vi "ParseRealTimeData.vi"(8 "error in (no error)":errorcluster, 11 "Raw Data":string) -> (0 "error out":errorcluster, 2 "BuySellBar":cluster{dbl[], dbl[]}[](graph), 3 "Price":T1)   [LabVIEW 2013]
uses:
  ctrl/TYPE Price.ctl
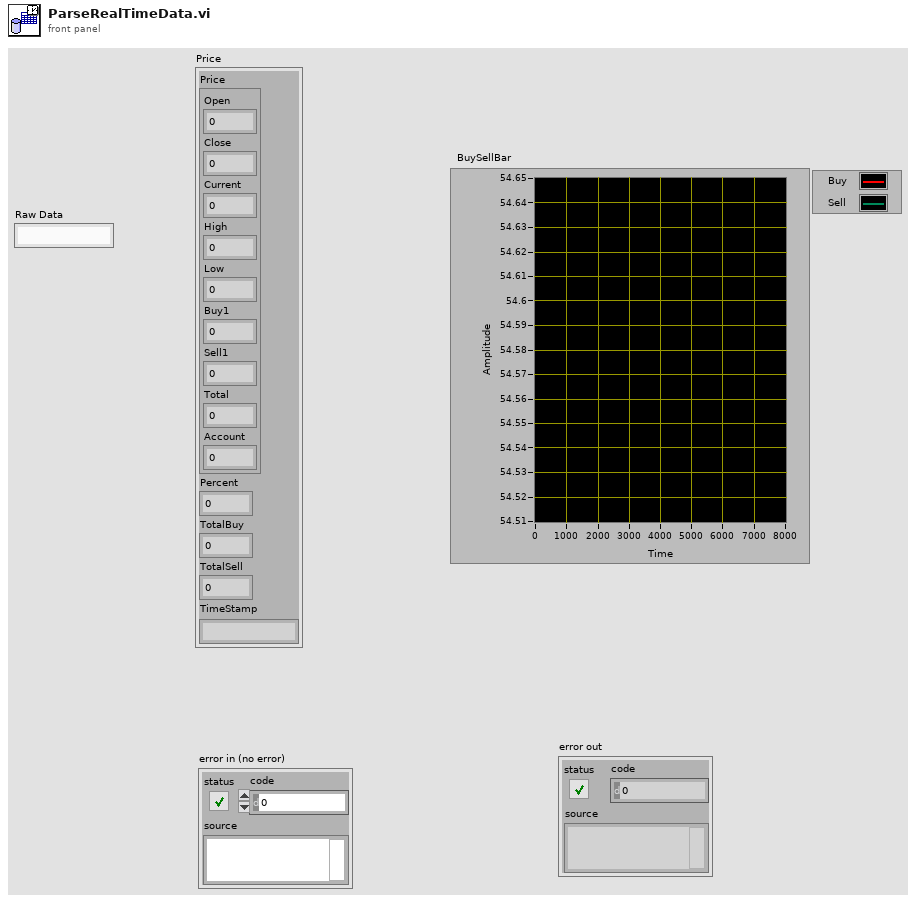
[diagram p1: front panel]
types:
  T1 = typedef "TYPE Price.ctl" = cluster{"Price":cluster{"Open":dbl, "Close":dbl, "Current":dbl, "High":dbl, "Low":dbl, "Buy1":dbl, "Sell1":dbl, "Total":dbl, "Account":dbl}, "Percent":dbl, "TotalBuy":dbl, "TotalSell":dbl, "TimeStamp":string}
  T2 = cluster{"[0]":dbl, "[1]":dbl, "[2]":dbl, "[3]":dbl, "[4]":dbl, "[5]":dbl, "[6]":dbl, "[7]":dbl, "[8]":dbl}
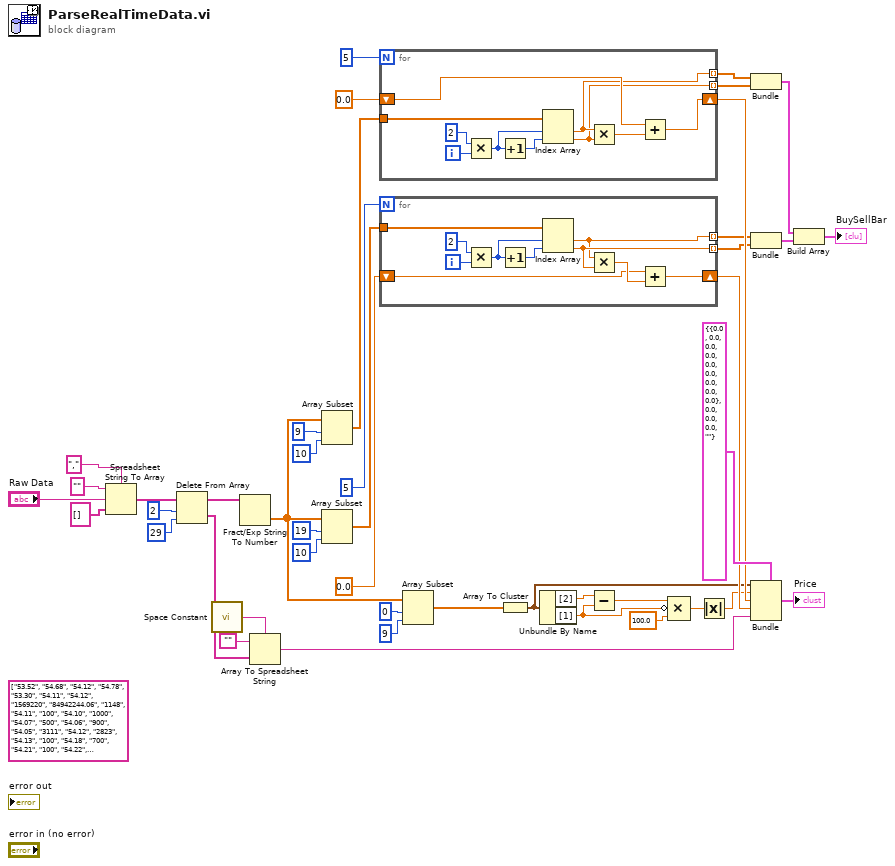
[diagram p0: block diagram]
diagram:
  (unwired) string[] ["53.52", "54.68", "54.12", "54.78", "53.30", "54.11", "54.12", "1569220", "84942244.06", "1148", "54.11", "100", "54.10", "1000", "54.07", "500", "54.06", "900", "54.05", "3111", "54.12", "2823", "54.13", "100", "54.18", "700", "54.21", "100", "54.22", "2014-05-21", "11:05:03", "00"] ("Data")
  n1 = Spreadsheet String To Array(delimiter (Tab)=",", format string="", spreadsheet string="Raw Data", array type (2D Dbl)=string[] []) -> (array=w9:string[])
  n2 = Delete From Array(array=w9, length=2, index=29) -> (deleted portion=w38:string[], array with subset deleted=w35:string[])
  n3 = call <vilib>:"Space Constant.vi"() -> ("String"=w36:string)
  n4 = Fract/Exp String To Number(string=w35) -> (number=w28:dbl[])  [unwired: 3 in, 1 out]
  n5 = Array To Spreadsheet String(delimiter (Tab)=w36, array=w38, 3:"" ("format string")) -> (spreadsheet string=w4:string)
  n6 = Array Subset(array=w28, index=9, length=10) -> (w25:dbl[])
  n7 = Array Subset(array=w28, index=19, length=10) -> (w22:dbl[])
  n8 = for {
    N: 5 -> [_]
    tunnel: w25 -> [w54]
    shift-right: [w48] -> w18
    shift-left: 0.0 -> [w47]
    tunnel: [w46] -> w13 mode=indexing
    tunnel: [w45] -> w12 mode=indexing
    i -> [w53]
    n9 = Multiply(x=2, y=w53) -> (x*y=w51:i32)
    n10 = Increment(x=w51) -> (x+1=w52:i32)
    n11 = Index Array(array=w54, index #1=w51, index #2=w52) -> (element #1=w46:dbl, element #2=w45:dbl)
    n12 = Multiply(x=w46, y=w45) -> (x*y=w49:dbl)
    n13 = Add(x=w47, y=w49) -> (x+y=w48:dbl)
  }
  n14 = for {
    N: 5 -> [_]
    tunnel: w22 -> [w64]
    shift-right: [w58] -> w17
    shift-left: 0.0 -> [w57]
    tunnel: [w56] -> w10 mode=indexing
    tunnel: [w55] -> w11 mode=indexing
    i -> [w63]
    n15 = Multiply(x=2, y=w63) -> (x*y=w61:i32)
    n16 = Increment(x=w61) -> (x+1=w62:i32)
    n17 = Index Array(array=w64, index #1=w61, index #2=w62) -> (element #1=w55:dbl, element #2=w56:dbl)
    n18 = Multiply(x=w55, y=w56) -> (x*y=w59:dbl)
    n19 = Add(x=w57, y=w59) -> (x+y=w58:dbl)
  }
  n20 = Array Subset(array=w28, index=0, length=9) -> (w27:dbl[])
  n21 = Array To Cluster(array=w27) -> (cluster=w8:T2)
  n22 = Unbundle By Name(w8) -> ("[2]"=w7:dbl, "[1]"=w5:dbl)
  n23 = Subtract(x=w7, y=w5) -> (x-y=w6:dbl)
  n24 = Compound Arithmetic op=MULTIPLY(w6, invert w5, 100.0 ("value")) -> (w3:dbl)
  n25 = Absolute Value(x=w3) -> (abs(x)=w1:dbl)
  n26 = Bundle(w13, w12) -> (w16:cluster{dbl[], dbl[]})  [unwired: 1 in]
  n27 = Bundle(w11, w10) -> (w15:cluster{dbl[], dbl[]})  [unwired: 1 in]
  n28 = Bundle(cluster=T1 {"Price"={"Open"=0.0, "Close"=0.0, "Current"=0.0, "High"=0.0, "Low"=0.0, "Buy1"=0.0, "Sell1"=0.0, "Total"=0.0, "Account"=0.0}, "Percent"=0.0, "TotalBuy"=0.0, "TotalSell"=0.0, "TimeStamp"=""}, "Price"=w8, "Percent"=w1, "TotalBuy"=w18, "TotalSell"=w17, "TimeStamp"=w4) -> (→"Price":T1)
  n29 = Build Array(w16, w15) -> (→"BuySellBar":cluster{dbl[], dbl[]}[])
